vi "Constructor.vi"(11 "Decaf in":refnum<class "Decaf.lvclass">) -> (3 "Decaf out":refnum<class "Decaf.lvclass">)   [LabVIEW 2011, in "Decaf.lvclass"]
uses:
  Decaf.lvclass
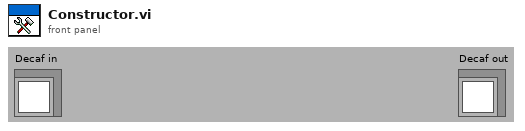
[diagram p1: front panel]
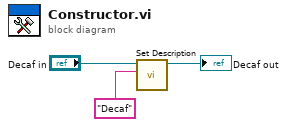
[diagram p0: block diagram]
diagram:
  n1 = call-dynamic "Set Description.vi"("Description"="Decaf", "Beverage in"="Decaf in") -> ("Beverage out"=→"Decaf out":refnum<class "Decaf.lvclass">)  [unwired: 9 in]
